vi "Dail LH_Barcode read.vi"(8 "error in":errorcluster, 11 "queue in":refnum<queue>) -> (0 "error out":errorcluster, 1 "exit":bool, 2 "read buffer":string, 3 "queue Out 2":refnum<queue>)   [LabVIEW 2015]
uses:
  Test  enqueue/AutoTest seq.ctl
  <vilib>/Instr/_visa.llb/VISA Configure Serial Port (Instr).vi
  Galobal variable_TI.vi
  Project Setup/Globle Variable/GR_Servo.vi
panel:
  out "x = y?":bool
  out "substring":string
  out "error out 2":errorcluster
  out "error out":errorcluster
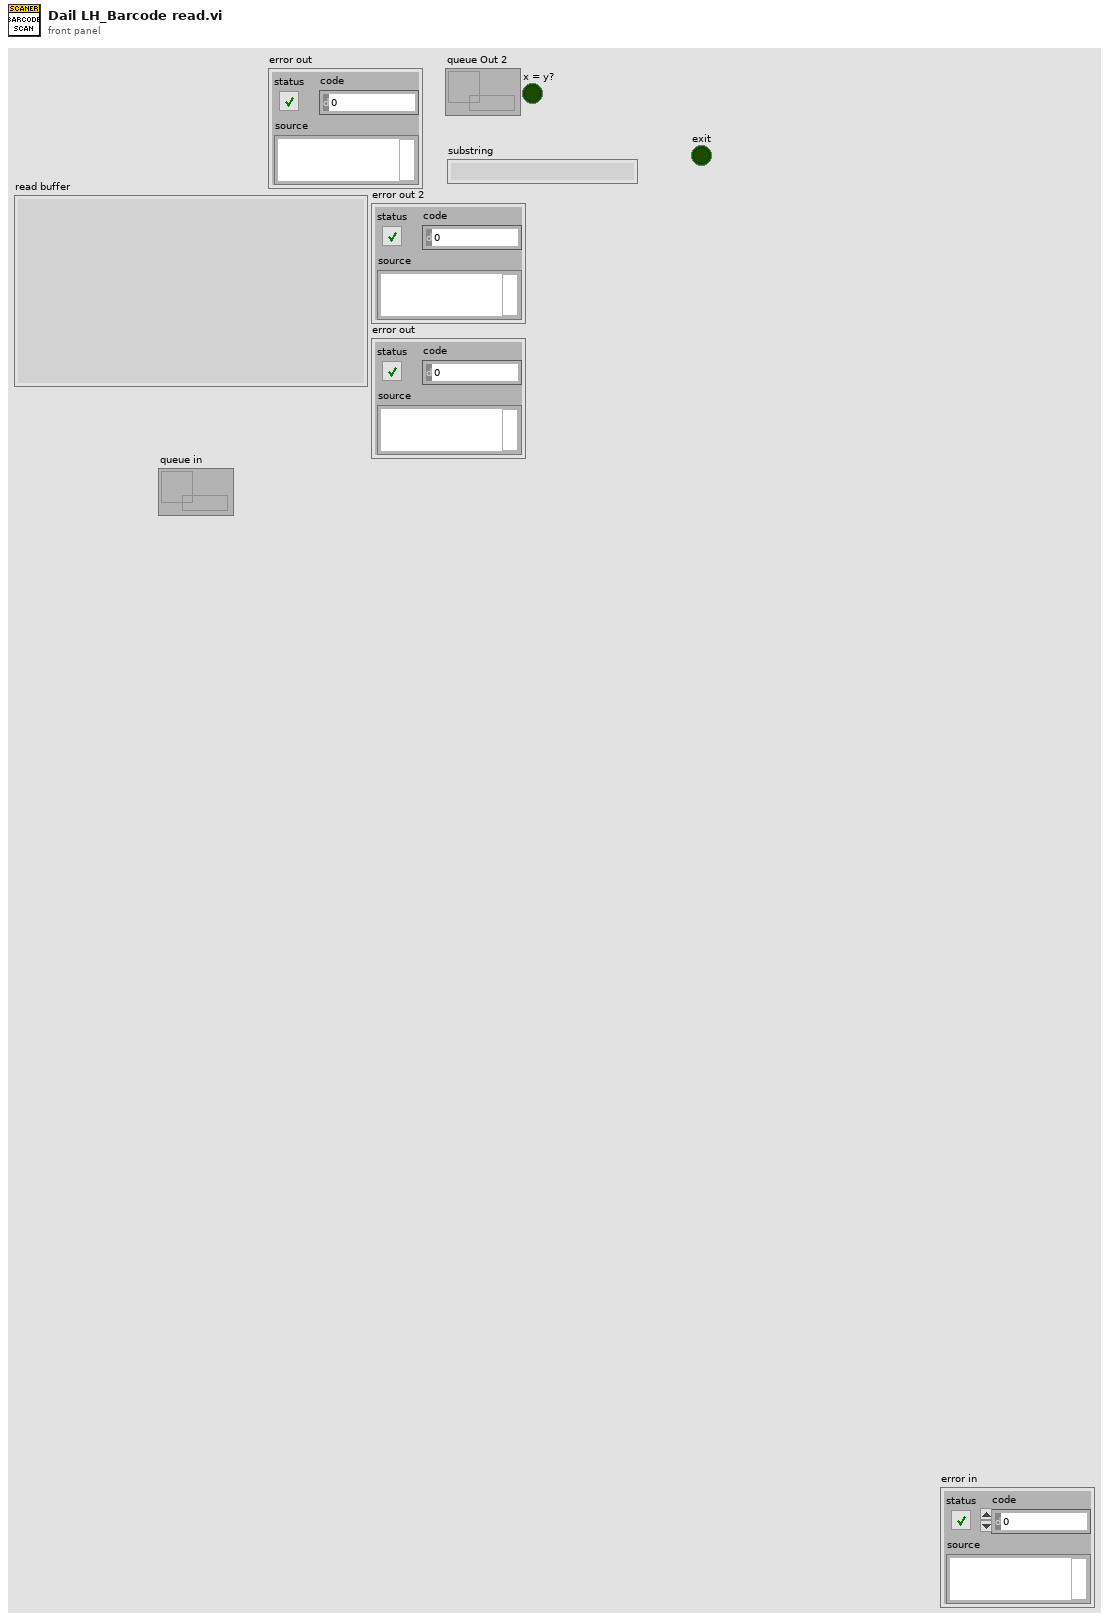
[diagram p1: front panel]
types:
  T1 = cluster{"MaxLoad(N) ":dbl, "Min Load(N)":dbl, "Load Offset":dbl, "Model":string, "MIC Code":string, "Dial Speedo":string, "Dial RMP":string, "Blinker":string, "Telltale":string}
  T2 = cluster{"Start":bool, "Emergency ":bool, "Reset":bool, "Home":bool, "Safety":bool}
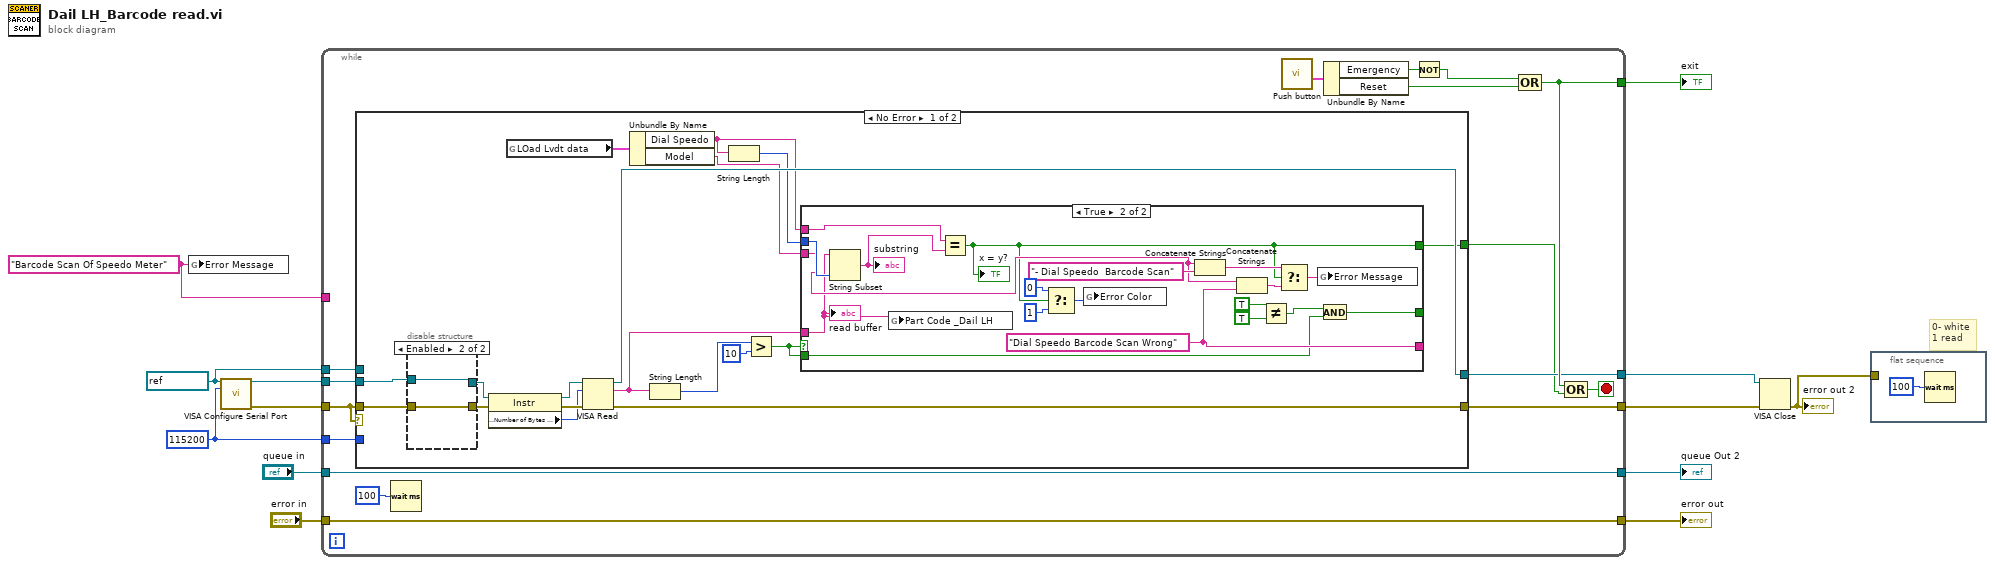
[diagram p0: block diagram]
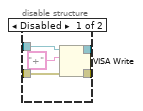
[diagram p2: hidden frame]
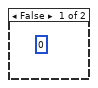
[diagram p3: hidden frame]
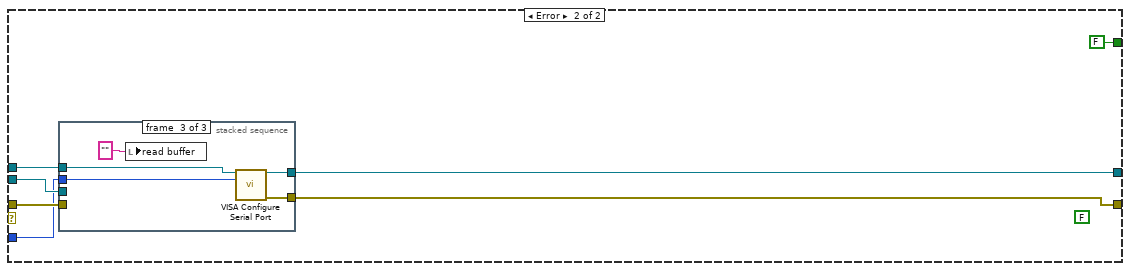
[diagram p4: hidden frame]
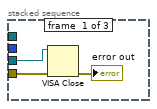
[diagram p5: hidden frame]
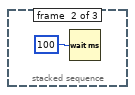
[diagram p6: hidden frame]
diagram:
  w1 = "Barcode Scan Of Speedo Meter" ("Error Message")
  w8 = u32 115200 ("baud rate (9600)")
  w9 = refnum<visa-resource-name> "COM2" ("VISA resource name")
  # "0- white\n1 read"
  n1 = global write "GR_Servo.vi" "Error Message"(w1) -> ()
  n2 = call-poly "VISA Configure Serial Port"("VISA resource name"=w9, "baud rate (9600)"=w8) -> ("VISA resource name out"=w13:refnum<visa-resource-name>, "error out"=w12:errorcluster)  [unwired: 12 in]
  n3 = while {
    tunnel: w13 -> [w29]
    tunnel: w12 -> [w27]
    tunnel: [w15] -> w11
    tunnel: [w28] -> w10
    tunnel: w9 -> [w26]
    tunnel: w8 -> [w25]
    tunnel: [w16] -> w7
    tunnel: [w22] -> w5
    tunnel: "queue in" -> [w22]
    tunnel: "error in" -> [w21]
    tunnel: [w21] -> w3
    tunnel: w1 -> [_]
    stop <- w23 stop-if-true
    n4 = case shown="No Error" w27 {
      tunnel: w29 -> [w47 w80]
      tunnel: w27 -> [w46 w79]
      tunnel: [w45 w76] -> w15
      tunnel: [w44 w75] -> w28
      tunnel: w26 -> [_ w78]
      tunnel: w25 -> [_ w77]
      tunnel: [w31 FALSE] -> w14
      frame No Error {
        n5 = disable-structure shown="Enabled" {
          disable-tunnel: w47 -> [w52 w54]
          disable-tunnel: w46 -> [w51 w53]
          disable-tunnel: [w50 w53] -> w43
          disable-tunnel: [w49 w54] -> w42
          frame Disabled {
            n6 = VISA Write(VISA resource name=w52, write buffer="+", error in (no error)=w51) -> (VISA resource name out=w49:refnum<visa-resource-name>, error out=w50:errorcluster)  [unwired: 1 out]
          }
          frame Enabled {
          }
        }
        n7 = property class="Instr"(reference=w42, error in=w43) -> (reference out=w41:refnum<visa-resource-name>, error out=w40:errorcluster, "Serial Settings:Number of Bytes at Serial Port"=w39:u32)
        n8 = global read "Galobal variable_TI.vi" "LOad Lvdt data"() -> (w35:T1)
        n9 = VISA Read(VISA resource name=w41, byte count=w39, error in (no error)=w40) -> (VISA resource name out=w45:refnum<visa-resource-name>, read buffer=w36:string, error out=w44:errorcluster)  [unwired: 1 out]
        n10 = Unbundle By Name(w35) -> ("Dial Speedo"=w34:string, "Model"=w32:string)
        n11 = String Length(string=w36) -> (length=w38:i32)
        n12 = String Length(string=w34) -> (length=w33:i32)
        n13 = Greater?(x=w38, y=10) -> (0:w30:bool)
        n14 = case shown="True" w30 {
          tunnel: w36 -> [_ w55]
          tunnel: w34 -> [_ w72]
          tunnel: w33 -> [_ w73]
          tunnel: w32 -> [_ w62]
          tunnel: [_ w61] -> w31
          tunnel: [_ w63] -> _
          tunnel: w30 -> [_ w58]
          tunnel: [_ w57] -> _
          frame False {
            (unwired) 0 ("f")
          }
          frame True {
            w63 = "Dial Speedo Barcode Scan Wrong" ("string")
            n15 = String Subset(string=w55, length (rest)=w73) -> (substring=w71:string)  [unwired: 1 in]
            "substring" <- w71
            n16 = global write "Galobal variable_TI.vi" "Part Code _Dail LH"(w55) -> ()
            n17 = Equal?(x=w72, y=w71) -> (x = y?=w61:bool)
            "x = y?" <- w61
            n18 = Select(t=0, s=w61, f=1) -> (s? t:f=w68:i32)
            n19 = global write "GR_Servo.vi" "Error Color"(w68) -> ()
            n20 = Concatenate Strings(w62, "- Dial Speedo  Barcode Scan" ("string")) -> (w66:string)
            n21 = Concatenate Strings(w62, w63) -> (w65:string)
            n22 = Not Equal?(x=TRUE, y=TRUE) -> (x != y?=w59:bool)
            n23 = Select(t=w66, s=w61, f=w65) -> (s? t:f=w64:string)
            n24 = global write "GR_Servo.vi" "Error Message"(w64) -> ()
            n25 = And(x=w59, y=w58) -> (x .and. y?=w57:bool)
            "read buffer" <- w55
          }
        }
      }
      frame Error {
        (unwired) FALSE
        n26 = stacked-sequence {
          tunnel: w80 -> [w82 _ _]
          tunnel: w79 -> [w81 _ _]
          tunnel: w78 -> [_ _ w89]
          tunnel: w77 -> [_ _ w88]
          tunnel: [_ _ w87] -> w76
          tunnel: [_ _ w86] -> w75
          frame #0 {
            n27 = VISA Close(VISA resource name=w82, error in (no error)=w81) -> (error out=→"error out":errorcluster)
          }
          frame #1 {
            n28 = Wait (ms)(milliseconds to wait=u32 100) -> ()  [unwired: 1 out]
          }
          frame #2 {
            n29 = local write "read buffer"("" ("read buffer")) -> ()
            n30 = call-poly "VISA Configure Serial Port"("VISA resource name"=w89, "baud rate (9600)"=w88) -> ("VISA resource name out"=w87:refnum<visa-resource-name>, "error out"=w86:errorcluster)  [unwired: 12 in]
          }
        }
      }
    }
    n31 = Wait (ms)(milliseconds to wait=u32 100) -> ()  [unwired: 1 out]
    n32 = call "Push button.vi"() -> ("Push Button"=w20:T2)  [unwired: 9 in, 2 out]
    n33 = Unbundle By Name(w20) -> ("Emergency"=w19:bool, "Reset"=w17:bool)
    n34 = Not(x=w19) -> (.not. x?=w18:bool)
    n35 = Compound Arithmetic op=OR(w18, w17) -> (w16:bool)
    n36 = Compound Arithmetic op=OR(w16, w14) -> (w23:bool)
  }
  "exit" <- w7
  "queue Out 2" <- w5
  "error out" <- w3
  n37 = VISA Close(VISA resource name=w11, error in (no error)=w10) -> (error out=w2:errorcluster)
  "error out 2" <- w2
  n38 = flat-sequence {
    tunnel: w2 -> [_]
    frame #0 {
      n39 = Wait (ms)(milliseconds to wait=u32 100) -> ()  [unwired: 1 out]
    }
  }
